vi "Dashboard Main.vi"() -> ()   [LabVIEW 2012]
uses:
  <vilib>/event_ctls.llb/eventvkey.ctl
  <vilib>/Utility/config.llb/Read Key (String).vi
  <vilib>/Utility/config.llb/Read Key (I32).vi
  <vilib>/Utility/config.llb/Write Key (String).vi
  <vilib>/Utility/config.llb/Write Key (I32).vi
  <vilib>/Utility/config.llb/NI_LVConfig.lvlib
  <vilib>/vision/NI_Vision_Development_Module.lvlib
panel:
  out "Battery Value":dbl(slide) scale=0.0..14.0 scale format="%#_2e"
  out "Battery":sgl(graph)
  in  "Camera Settings":T1={"Frate Rate"=30, "Compression"=30, "Size"=1} {"Frate Rate" scale=1.0..30.0; "Size" items=["640x480", "320x240", "160x120"]}
  out "Mode":T2(ring)=enum."Auto Disabled"
  out "Camera IP":string
  out "JS1 Z":dbl(slide) scale=-1.0..1.0 scale format="%#_2e"
  out "JS2 Z":dbl(slide) scale=-1.0..1.0 scale format="%#_2e"
  out "Joystick 1":cluster{"X":dbl, "Y":dbl}[](graph)
  out "Joystick 2":cluster{"X":dbl, "Y":dbl}[](graph)
  out "JS Buttons 1":T3
  out "JS Buttons 2":T3
  out "MotorSlide4":dbl(slide) scale=-1.0..1.0 scale format="%#_2e"
  out "MotorSlide3":dbl(slide) scale=-1.0..1.0 scale format="%#_2e"
  out "MotorSlide2":dbl(slide) scale=-1.0..1.0 scale format="%#_2e"
  in  "MotorName3":string="Front Left"
  in  "MotorName4":string="Front Right"
  in  "MotorName1":string="Rear Left"
  in  "MotorName2":string="Rear Right"
  out "MotorChart4":dbl(graph)
  out "MotorChart3":dbl(graph)
  out "MotorChart2":dbl(graph)
  out "MotorSlide1":dbl(slide) scale=-1.0..1.0 scale format="%#_2e"
  out "MotorChart1":dbl(graph)
  out "Robot IP":string
  in  "Dashboard Tab":enum32{"Operation", "Test", "Checklist"}(tab)
  in  "Checkbox 2":bool
  in  "Checkbox 1":bool
  in  "Slider 1":dbl(slide) scale=0.0..100.0
  in  "Slider":dbl(slide) scale=0.0..100.0 scale format="%#_3g"
  in  "On/Off":bool caption="Solenoid"
  in  "Test Name":u16(ring) items=["Select the test to run...", "Example Test", "-------------------------------", "List of tests is built in robot code.", "Replace with your own automated tests."]
  in  "Test Tree":string(tree)
  in  "Motor":cluster{"Value":dbl, "Enable":bool} {"Value" scale=-1.0..1.0 scale format="%#_3g"}
  out "Progress":T4 {"Test Progress" scale=0.0..100.0}
  in  "Rev/Fwd":cluster{"Forward":bool, "Reverse":bool}
  in  "Ring":u16(ring) items=["Auto", "Fixed indoor", "Fixed outdoor 1", "Fixed outdoor 2", "Fixed fluorescent 1", "Fixed fluorescent 2", "Hold current"]
  in  "Listbox":i32(listbox)
  in  "Viewer":T5(tab)
  out "Mbps":dbl format="%#.1g"
  in  "Enable":bool=TRUE
  in  "DB Camera Config":bool
  out "Mbps":bool
  out "fps":dbl format="%#.1g"
  out "Image Error Message":string="Timeout in Camera Communications"
  out "Camera Image":T6(plugin-control)
  out "Buttons 1":cluster{"1":bool, "2":bool, "3":bool}
  out "Kinect 1":cluster{"X":dbl, "Y":dbl, "Z":dbl} {"X" scale=1.0..-1.0; "Y" scale=1.0..-1.0; "Z" scale=1.0..-1.0}
  out "Buttons 2":cluster{"1":bool, "2":bool, "3":bool}
  out "Kinect 2":cluster{"X":dbl, "Y":dbl, "Z":dbl} {"X" scale=1.0..-1.0; "Y" scale=1.0..-1.0; "Z" scale=1.0..-1.0}
  out "Version":string
  out "Skeleton Picture":picture
  out "Players":i8
  out "Tree":string(tree)
  # "Drive & Motors"
  # "Robot IP:"
  # "Customize by placing controls and indicators here and name to match\nDashboard Variables on robot."
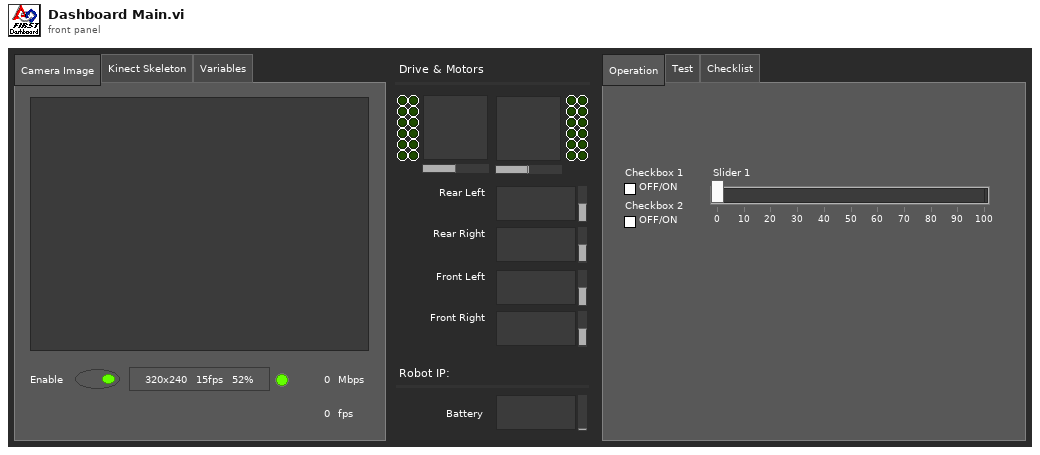
[diagram p1: front panel]
types:
  T1 = cluster{"Frate Rate":i32, "Compression":i32, "Size":u16}
  T2 = enum8{"Tele-Op Disabled", "Tele-Op Enabled", "Auto Disabled", "Auto Enabled", "Test Disabled", "Test Enabled", ""}
  T3 = cluster{bool, bool, bool, bool, bool, bool, bool, bool, bool, bool, bool, bool}
  T4 = cluster{"Test Progress":u8, "Test Progress Text":string}
  T5 = enum32{"Camera Image", "Kinect Skeleton", "Variables"}
  T6 = typedef "IMAQ Image.ctl" = refnum<image>
  T7 = typedef "Image Type" = u32
  T8 = typedef "LVBoundsTypeDef.ctl" = cluster{"Width":u32, "Height":u32}
  T9 = typedef "SkeletonTrackState.ctl" = enum32{"NotTracked", "PositionOnly", "Tracked"}
  T10 = cluster{"TrackingState":u8[], "Position":cluster{"x":sgl, "y":sgl, "z":sgl}, cluster{"x":sgl, "y":sgl, "z":sgl, sgl}[], "TrackState":T9}
  T11 = cluster{cluster{"ScaledToPercentRange":dbl, "ScaledToPercentRange":dbl, "ScaledToPercentRange":dbl}, cluster{bool, bool, bool}}[]
  T12 = cluster{cluster{"ScaledToPercentRange":dbl, "ScaledToPercentRange":dbl, "ScaledToPercentRange":dbl}, cluster{bool, bool, bool}}
  T13 = cluster{"ScaledToPercentRange":dbl, "ScaledToPercentRange":dbl, "ScaledToPercentRange":dbl}
  T14 = typedef "LVRectTypeDef.ctl" = cluster{"Left":i16, "Top":i16, "Right":i16, "Bottom":i16}
  T15 = cluster{"Competition mode":bool, "Robot Link":bool, "Autonomous":bool, "Enabled":bool, "E-Stop":bool, "Simulated":bool, "TestMode":bool, "Docked Window":bool}
  T16 = cluster{"Boolean Array[0]":bool, "Boolean Array[1]":bool, "Boolean Array[2]":bool, "Boolean Array[3]":bool, "Boolean Array[4]":bool, "Boolean Array[5]":bool, "Boolean Array[6]":bool, "Boolean Array[7]":bool, "Boolean Array[8]":bool, "Boolean Array[9]":bool, "Boolean Array[10]":bool, "Boolean Array[11]":bool}
  T17 = typedef "NI_LVConfig.lvlib/Config Data RefNum.ctl" = refnum<k1>
  T18 = typedef "eventvkey.ctl" = enum16{"ASCII", "Enter", "Return", "Shift", "Ctrl", "Alt", "Cmd", "Opt", "Caps", "NumLock", "Clear", "Break", "Up", "Down", "Left", "Right", "Insert", "Delete", "Home", "End", "PageUp", "PageDown", "Escape", "Help", "Pause", "ScrollLock", "F1", "F2", "F3", "F4", "F5", "F6", "F7", "F8", "F9", "F10", "F11", "F12", "F13", "F14", "F15", "F16", "F17", "F18", "F19", "F20", "F21", "F22", "F23", "F24", "Play", "VolumeUp", "VolumeDown", "Mute", "Two Byte Char"}
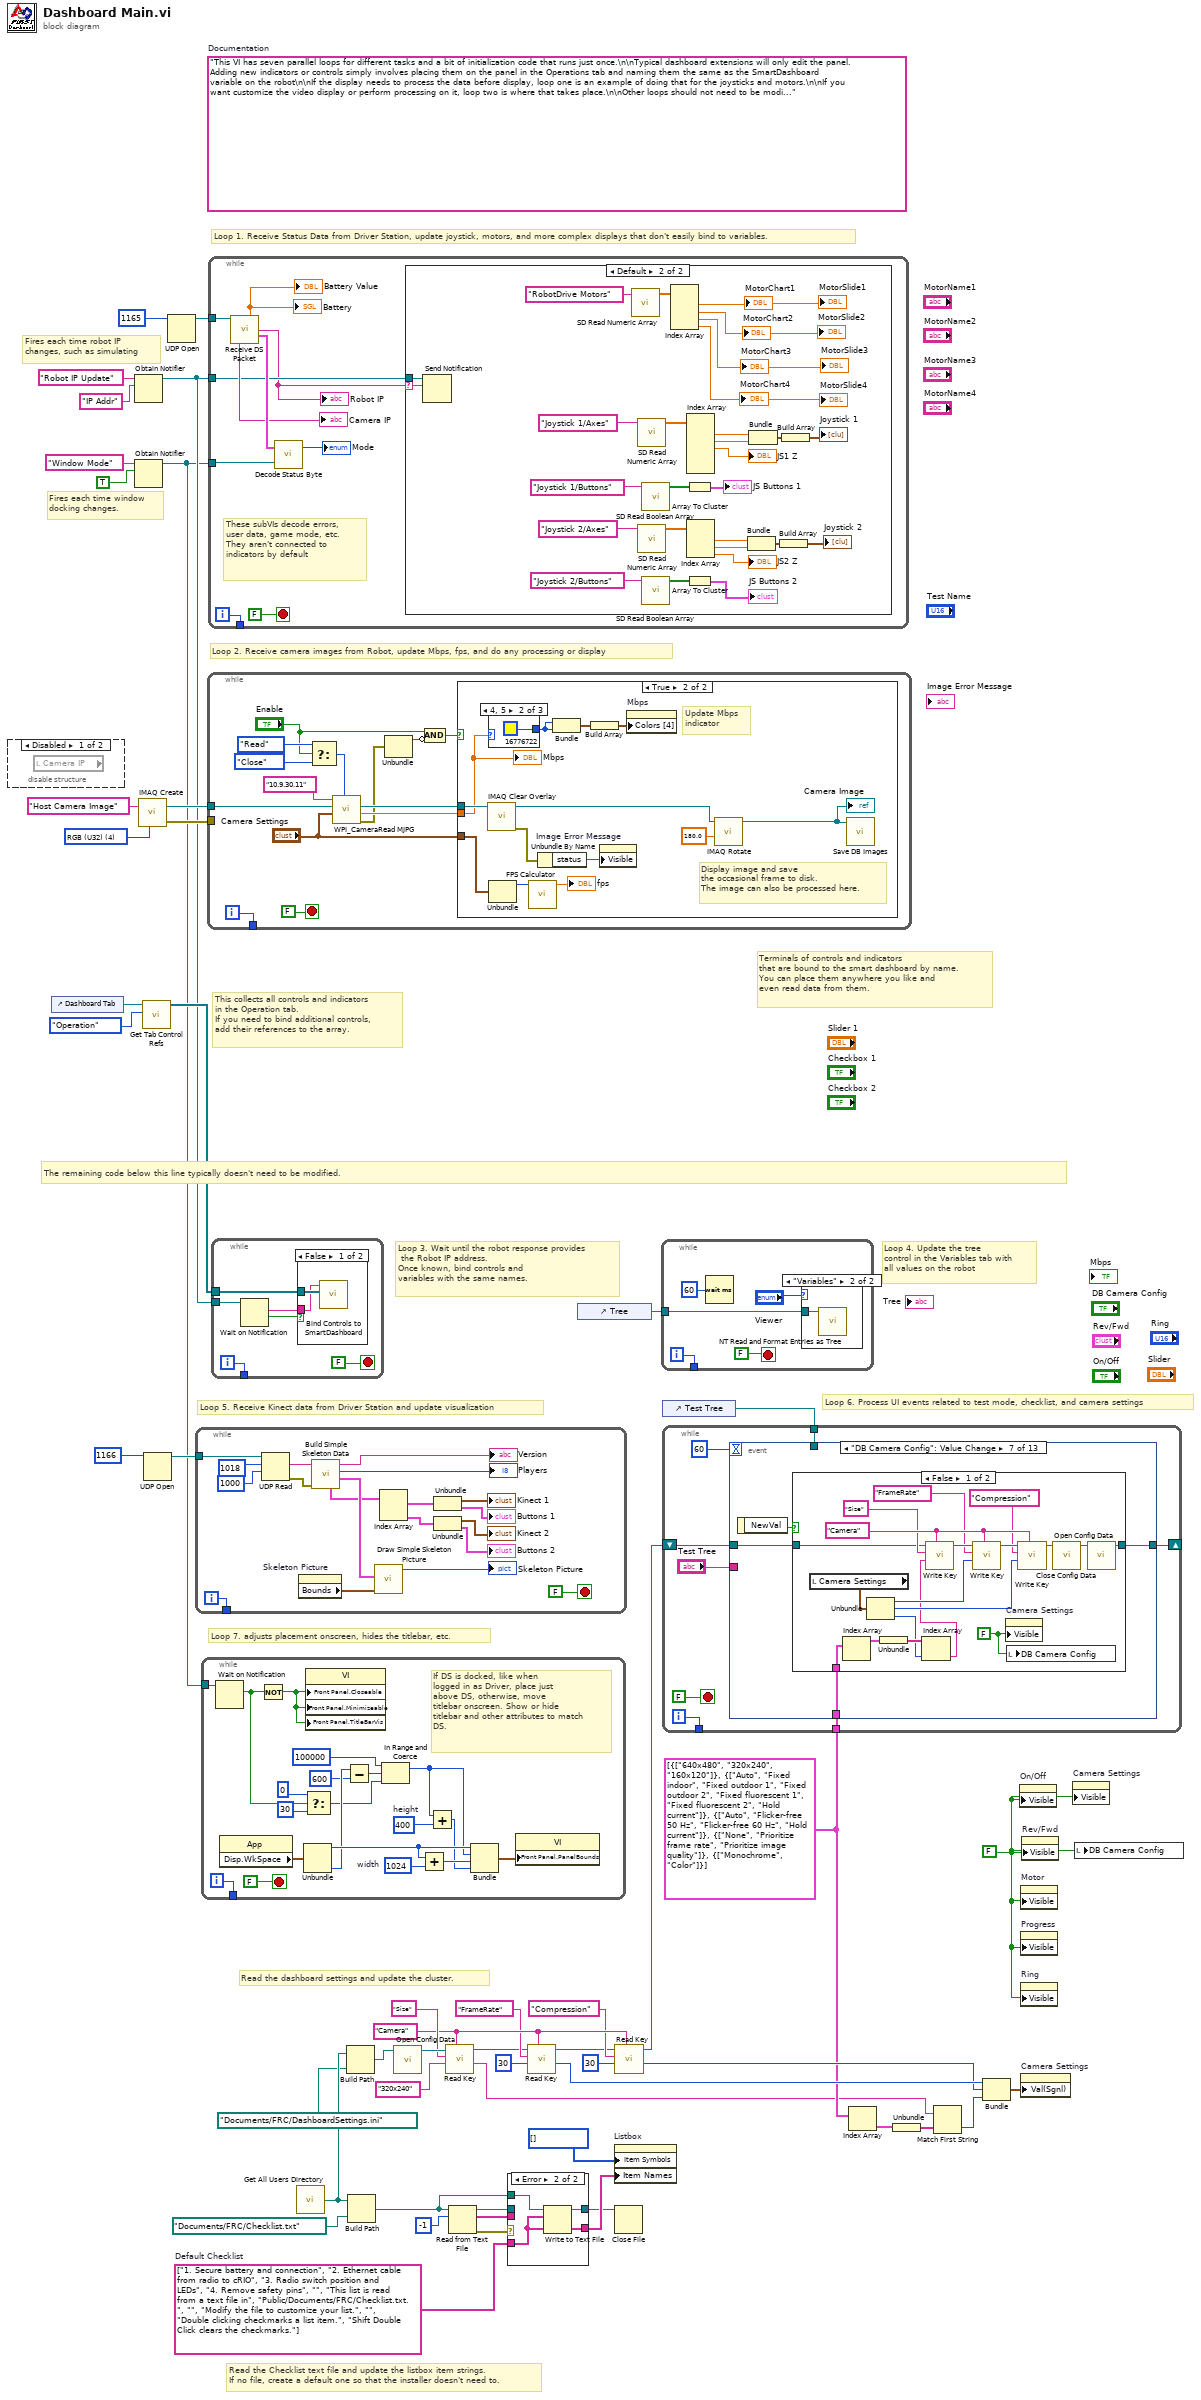
[diagram p0: block diagram]
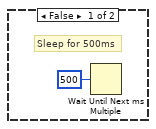
[diagram p4: hidden frame]
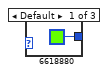
[diagram p5: hidden frame]
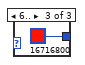
[diagram p6: hidden frame]
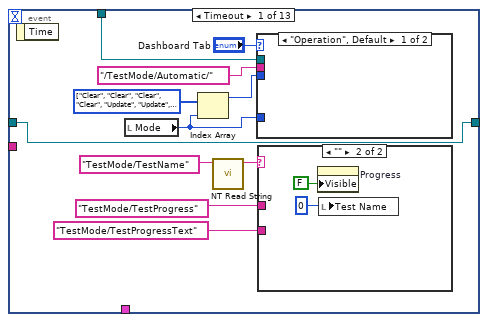
[diagram p8: hidden frame]
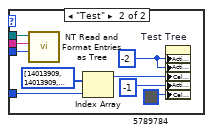
[diagram p9: hidden frame]
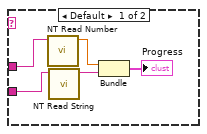
[diagram p10: hidden frame]
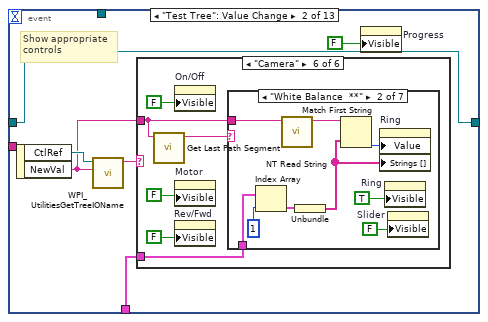
[diagram p11: hidden frame]
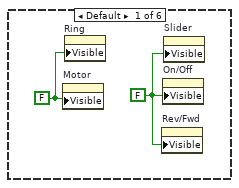
[diagram p12: hidden frame]
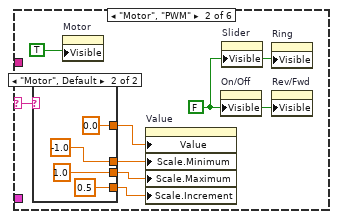
[diagram p13: hidden frame]
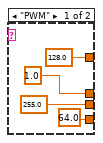
[diagram p14: hidden frame]
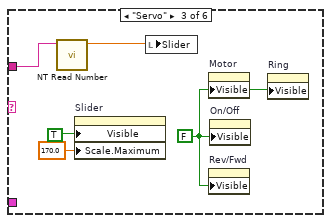
[diagram p15: hidden frame]
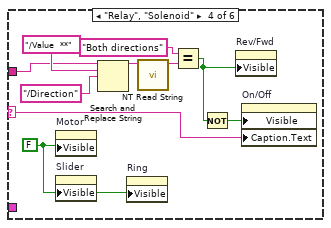
[diagram p16: hidden frame]
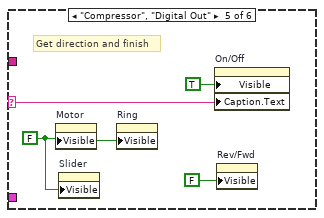
[diagram p17: hidden frame]
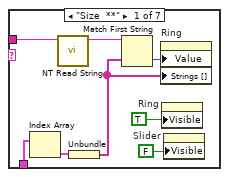
[diagram p18: hidden frame]
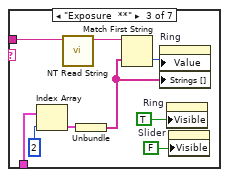
[diagram p19: hidden frame]
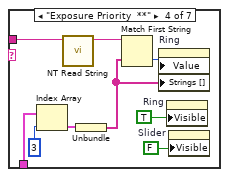
[diagram p20: hidden frame]
diagram:
  w21 = "Camera"
  w13 = cluster{string[]}[] [{["640x480", "320x240", "160x120"]}, {["Auto", "Fixed indoor", "Fixed outdoor 1", "Fixed outdoor 2", "Fixed fluorescent 1", "Fixed fluorescent 2", "Hold current"]}, {["Auto", "Flicker-free 50 Hz", "Flicker-free 60 Hz", "Hold current"]}, {["None", "Prioritize frame rate", "Prioritize image quality"]}, {["Monochrome", "Color"]}]
  w29 = string[] ["1. Secure battery and connection", "2. Ethernet cable from radio to cRIO", "3. Radio switch position and LEDs", "4. Remove safety pins", "", "This list is read from a text file in", "Public/Documents/FRC/Checklist.txt.", "", "Modify the file to customize your list.", "", "Double clicking checkmarks a list item.", "Shift Double Click clears the checkmarks."]  # Default Checklist
  w27 = FALSE ("Visible")
  (unwired) "This VI has seven parallel loops for different tasks and a bit of initialization code that runs just once.\n\nTypical dashboard extensions will only edit the panel. Adding new indicators or controls simply involves placing them on the panel in the Operations tab and naming them the same as the SmartDashboard variable on the robot\n\nIf the display needs to process the data before display, loop one is an example of doing that for the joysticks and motors.\n\nIf you want customize the video display or perform processing on it, loop two is where that takes place.\n\nOther loops should not need to be modified. They are pretty standard, and document the task they perform."  # Documentation
  w50 = T7 4 items=["Grayscale (U8)", "Grayscale (I16)", "Grayscale (SGL)", "Complex (CSG)", "RGB (U32)", "HSL (U32)", "RGB (U64)"] ("Image Type")
  # "Fires each time robot IP\nchanges, such as simulating"
  # "Fires each time window\ndocking changes."
  # "Read the Checklist text file and update the listbox item strings.\nIf no file, create a default one so that the installer doesn't need to."
  # "This collects all controls and indicators\nin the Operation tab.\nIf you need to bind additional controls,\nadd their references to the array."
  # "The remaining code below this line typically doesn't need to be modified."
  # "Loop 6. Process UI events related to test mode, checklist, and camera settings"
  # "Read the dashboard settings and update the cluster."
  # "Terminals of controls and indicators\nthat are bound to the smart dashboard by name.\nYou can place them anywhere you like and\neven read data from them."
  # "Loop 4. Update the tree\ncontrol in the Variables tab with\nall values on the robot"
  # "Loop 3. Wait until the robot response provides\n the Robot IP address.\nOnce known, bind controls and\nvariables with the same names."
  # "Loop 5. Receive Kinect data from Driver Station and update visualization"
  # "Loop 7. adjusts placement onscreen, hides the titlebar, etc."
  # "Loop 1. Receive Status Data from Driver Station, update joystick, motors, and more complex displays that don't easily bind to variables."
  # "Loop 2. Receive camera images from Robot, update Mbps, fps, and do any processing or display"
  n1 = disable-structure shown="Disabled" {
    frame Disabled {
      n2 = local read "Camera IP"() -> ()  [unwired: 1 out]
    }
    frame Enabled {
    }
  }
  n3 = control-ref of="Dashboard Tab"() -> (w43:refnum<vi>)
  n4 = Obtain Notifier(name (unnamed)="Robot IP Update", notification data type="IP Addr" ("name (unnamed)")) -> (notifier out=w40:refnum<notifier>)  [unwired: 2 in, 2 out]
  n5 = Obtain Notifier(name (unnamed)="Window Mode", notification data type=TRUE) -> (notifier out=w33:refnum<notifier>)  [unwired: 2 in, 2 out]
  n6 = call "IMAQ Create"("Image Name"="Host Camera Image", "Image Type"=w50) -> ("New Image"=w48:T6, "error out"=w47:errorcluster)  [unwired: 2 in, 1 out]
  n7 = call <vilib>:"Get Tab Control Refs.vi"("Page Index"=enum32{"Operation", "Test"}."Operation" ("Dashboard Tab"), "TabControl in"=w43) -> ("ControlsOnPage"=w44:refnum<vi>[])  [unwired: 9 in]
  n8 = UDP Open(11:u16 1166 ("port")) -> (port=w45:refnum<k16>)  [unwired: 2 in, 4 out]
  n9 = UDP Open(11:u16 1165 ("port")) -> (port=w51:refnum<k16>)  [unwired: 2 in, 4 out]
  n10 = while {
    tunnel: w45 -> [w69]
    tunnel: [w54] -> _
    i -> [w54]
    stop <- FALSE stop-if-true
    n11 = UDP Read(connection ID=w69, max size (548)=1018 ("bytes to read"), timeout ms (25000)=1000) -> (data out=w63:string, error out=w53:errorcluster)  [unwired: 1 in, 3 out]
    n12 = property on="Skeleton Picture" class="Pict"() -> ("Bounds"=w65:T8)  [unwired: 2 in, 2 out]
    n13 = call "Build Simple Skeleton Data.vi"("error in (no error)"=w53, "data in"=w63) -> ("Skeleton Data"=w64:T10, "NumPlayers"=→"Players":i8, "Version String"=→"Version":string, "Simple Joystick Info"=w61:T11)  [unwired: 5 in, 1 out]
    n14 = call "Draw Simple Skeleton Picture.vi"("Bounds"=w65, "Simple Skeleton"=w64) -> ("new picture out"=→"Skeleton Picture":picture)  [unwired: 9 in]
    n15 = Index Array(array=w61) -> (element #1=w60:T12, element #2=w59:T12)  [unwired: 2 in]
    n16 = Unbundle(w60) -> (→"Kinect 1":T13, →"Buttons 1":cluster{bool, bool, bool})
    n17 = Unbundle(w59) -> (→"Kinect 2":T13, →"Buttons 2":cluster{bool, bool, bool})
  }
  n18 = while {
    tunnel: w33 -> [w90]
    tunnel: [w88] -> _
    i -> [w88]
    stop <- FALSE stop-if-true
    w80 = 1024  # width
    w83 = 400  # height
    # "If DS is docked, like when\nlogged in as Driver, place just\nabove DS, otherwise, move\ntitlebar onscreen. Show or hide\ntitlebar and other attributes to match\nDS."
    n19 = Wait on Notification(notifier=w90) -> (notification=w75:bool)  [unwired: 3 in, 3 out]
    n20 = property class="App"() -> ("Disp.WkSpace"=w86:T14)  [unwired: 2 in, 2 out]
    n21 = Not(x=w75) -> (.not. x?=w89:bool)
    n22 = Unbundle(w86) -> ("Left"=w84:i16, "Bottom"=w81:i16)  [unwired: 2 out]
    n23 = Select(t=0, s=w75, f=30) -> (s? t:f=w74:i32)
    n24 = property class="VI"("Front Panel.Closeable"=w89, "Front Panel.Minimizeable"=w89, "Front Panel.TitleBarVis"=w89) -> ()  [unwired: 2 in, 2 out]
    n25 = Subtract(x=w81, y=600) -> (x-y=w78:i32)
    n26 = In Range and Coerce(upper limit=100000, x=w78, lower limit=w74) -> (coerced(x)=w72:i32)  [unwired: 1 out]
    n27 = Add(x=w84, y=w80) -> (x+y=w85:i32)
    n28 = Add(x=w72, y=w83) -> (x+y=w82:i32)
    n29 = Bundle("Left"=w84, w72, w85, w82) -> (w87:cluster{"Left":i16, i32, i32, i32})  [unwired: 1 out]
    n30 = property class="VI"("Front Panel.PanelBounds"=w87) -> ()  [unwired: 2 in, 2 out]
  }
  n31 = while {
    tunnel: w48 -> [w102]
    tunnel: w47 -> [_]
    tunnel: [w104] -> _
    i -> [w104]
    stop <- FALSE stop-if-true
    n32 = Select(t=enum16{"Read", "Reopen", "Close"}."Read" ("Operation"), s="Enable", f=enum16{"Read", "Reopen", "Close"}."Close" ("Operation")) -> (s? t:f=w97:enum16{"Read", "Reopen", "Close"})
    n33 = call <vilib>:"WPI_CameraRead MJPG.vi"("Operation"=w97, "Camera Settings"="Camera Settings", "Image"=w102, "address"="10.9.30.11") -> ("error out"=w96:errorcluster, "Bandwidth (kbps)"=w100:dbl, "Image Out"=w101:T6)  [unwired: 5 in]
    n34 = Unbundle(w96) -> ("status"=w94:bool)  [unwired: 2 out]
    n35 = Compound Arithmetic op=AND("Enable", invert w94) -> (w93:bool)
    n36 = case shown="True" w93 {
      tunnel: "Camera Settings" -> [_ w111]
      tunnel: w101 -> [_ w114]
      tunnel: w100 -> [_ w113]
      frame False {
        # "Sleep for 500ms"
        n37 = Wait Until Next ms Multiple(millisecond multiple=u32 500) -> ()  [unwired: 1 out]
      }
      frame True {
        # "Display image and save\nthe occasional frame to disk.\nThe image can also be processed here."
        # "Update Mbps\nindicator"
        n38 = call "IMAQ Clear Overlay"("Image"=w114) -> ("error out"=w118:errorcluster, "Image Out"=w109:T6)  [unwired: 2 in, 7 out]
        n39 = case shown="4, 5" w113 {
          tunnel: [u32 6618880 ("Color Box") u32 16776722 ("Color Box") u32 16716800 ("Color Box")] -> w115
          frame Default {
          }
          frame 4, 5 {
          }
          frame 6.. {
          }
        }
        n40 = Unbundle(w111) -> ("Frate Rate"=w110:i32)  [unwired: 2 out]
        n41 = call "FPS Calculator.vi"("Average Count"=w110) -> ("fps"=→"fps":dbl)  [unwired: 10 in]
        n42 = Unbundle By Name(w118) -> ("status"=w119:bool)
        n43 = Bundle("Color Box"=w115, "Color Box"=w115) -> (w117:cluster{"Color Box":u32, "Color Box":u32})  [unwired: 1 out]
        n44 = Build Array(w117) -> (w116:cluster{"Color Box":u32, "Color Box":u32}[])
        n45 = property on="Image Error Message" class="Str"("Visible"=w119) -> ()  [unwired: 2 in, 2 out]
        n46 = property on="Mbps" class="Bool (strict)"("Colors [4]"=w116) -> ()  [unwired: 2 in, 2 out]
        n47 = call "IMAQ Rotate"("Angle (degrees)"=sgl 180.0, "Image Src"=w109) -> ("Image Dst Out"=w107:T6)  [unwired: 8 in, 1 out]
        "Camera Image" <- w107
        n48 = call "Save DB Images.vi"("Image"=w107) -> ()  [unwired: 2 in, 1 out]
        "Mbps" <- w113
      }
    }
  }
  n49 = while {
    tunnel: w51 -> [w130]
    tunnel: w40 -> [w124]
    tunnel: w33 -> [w128]
    tunnel: [w125] -> _
    i -> [w125]
    stop <- FALSE stop-if-true
    # "These subVIs decode errors, user data, game mode, etc.\nThey aren't connected to indicators by default"
    n50 = call "Receive DS Packet.vi"("Recv Socket"=w130) -> ("Battery"=→"Battery" →"Battery Value":sgl, "Robot IP Address"=w123:string, "Status"=w131:T15, "Camera IP Address"=→"Camera IP":string)  [unwired: 1 in, 10 out]
    "Robot IP" <- w123
    n51 = call "Decode Status Byte.vi"("Window Mode Notifier"=w128, "Status"=w131) -> ("Mode"=→"Mode":T2)  [unwired: 1 out]
    n52 = case shown="Default" w123 {
      selector: w123 -> [_ w133]
      tunnel: w124 -> [_ w134]
      frame "0.0.0.0" {
        # "Robot not responding, don't poll the variables"
      }
      frame Default {
        n53 = Send Notification(notification=w133, notifier=w134) -> ()  [unwired: 1 in, 2 out]
        n54 = call <vilib>:"SD Read Numeric Array.vi"("Name"="RobotDrive Motors") -> ("Numeric Array"=w157:dbl[])  [unwired: 8 in, 2 out]
        n55 = call <vilib>:"SD Read Numeric Array.vi"("Name"="Joystick 1/Axes") -> ("Numeric Array"=w150:dbl[])  [unwired: 8 in, 2 out]
        n56 = call <vilib>:"SD Read Numeric Array.vi"("Name"="Joystick 2/Axes") -> ("Numeric Array"=w144:dbl[])  [unwired: 8 in, 2 out]
        n57 = call <vilib>:"SD Read Boolean Array.vi"("Name"="Joystick 1/Buttons") -> ("Boolean Array"=w152:bool[])  [unwired: 8 in, 2 out]
        n58 = call <vilib>:"SD Read Boolean Array.vi"("Name"="Joystick 2/Buttons") -> ("Boolean Array"=w143:bool[])  [unwired: 8 in, 2 out]
        n59 = Index Array(array=w157) -> (element #1=→"MotorChart1" →"MotorSlide1":dbl, element #2=→"MotorSlide2" →"MotorChart2":dbl, element #3=→"MotorChart3" →"MotorSlide3":dbl, element #4=→"MotorChart4" →"MotorSlide4":dbl)  [unwired: 4 in]
        n60 = Array To Cluster(array=w152) -> (cluster=→"JS Buttons 1":T16)
        n61 = Array To Cluster(array=w143) -> (cluster=→"JS Buttons 2":T16)
        n62 = Index Array(array=w150) -> (element #1=w147:dbl, element #2=w148:dbl, element #3=→"JS1 Z":dbl)  [unwired: 6 in, 3 out]
        n63 = Index Array(array=w144) -> (element #1=w139:dbl, element #2=w138:dbl, element #3=→"JS2 Z":dbl)  [unwired: 3 in]
        n64 = Bundle("Numeric"=w139, "Numeric"=w138) -> (w140:cluster{"Numeric":dbl, "Numeric":dbl})  [unwired: 1 in]
        n65 = Bundle("Numeric"=w147, "Numeric"=w148) -> (w146:cluster{"Numeric":dbl, "Numeric":dbl})  [unwired: 1 in]
        n66 = Build Array(w140) -> (→"Joystick 2":cluster{"Numeric":dbl, "Numeric":dbl}[])
        n67 = Build Array(w146) -> (→"Joystick 1":cluster{"Numeric":dbl, "Numeric":dbl}[])
      }
    }
  }
  n68 = while {
    tunnel: w44 -> [w166]
    tunnel: w40 -> [w163]
    tunnel: [w161] -> _
    i -> [w161]
    stop <- FALSE stop-if-true
    n69 = Wait on Notification(notifier=w163) -> (notification=w162:string, timed out?=w164:bool)  [unwired: 3 in, 2 out]
    n70 = case shown="False" w164 {
      tunnel: w166 -> [w168 _]
      tunnel: w162 -> [w167 _]
      frame False {
        n71 = call <vilib>:"Bind Controls to SmartDashboard.vi"("Bound Control Refs"=w168, "Server IP Address"=w167) -> ()  [unwired: 10 in]
      }
      frame True {
      }
    }
  }
  n72 = call "Get All Users Directory.vi"() -> ("All User Path"=w26:path)
  n73 = Build Path(base path=w26, name or relative path=path "Documents/FRC/DashboardSettings.ini") -> (appended path=w25:path)
  n74 = Build Path(base path=w26, name or relative path=path "Documents/FRC/Checklist.txt") -> (appended path=w30:path)
  n75 = call <vilib>:"Open Config Data.vi"("configuration file path"=w25) -> ("refnum"=w24:T17)  [unwired: 8 in, 2 out]
  n76 = call-poly <vilib>:"Read Key.vi"("section"=w21, "default value"="320x240", "key"="Size", "refnum"=w24) -> ("value"=w11:string, "refnum out"=w6:T17)  [unwired: 2 in, 4 out]
  n77 = Read from Text File(file (use dialog)=w30, count=-1 ("timeout ms (25000)")) -> (refnum out=w8:refnum<file>, text=w31:string[], error out=w32:errorcluster)  [unwired: 2 in, 1 out]
  n78 = case shown="Error" w32 {
    tunnel: w31 -> [w170 _]
    tunnel: [w170 w172] -> w28
    tunnel: w29 -> [_ w172]
    tunnel: w30 -> [_ w173]
    tunnel: [w169 w171] -> w7
    tunnel: w8 -> [w169 _]
    frame No Error {
    }
    frame Error {
      n79 = Write to Text File(file (use dialog)=w173, text=w172) -> (refnum out=w171:refnum<file>)  [unwired: 2 in, 2 out]
    }
  }
  n80 = call-poly <vilib>:"Read Key.vi"("section"=w21, "default value"=30, "key"="FrameRate", "refnum"=w6) -> ("value"=w16:i32, "refnum out"=w5:T17)  [unwired: 1 in, 5 out]
  n81 = control-ref of="Tree"() -> (w2:refnum<vi>)
  n82 = property on="Listbox" class="LstBox (strict)"("Item Symbols"=i32[] [], "Item Names"=w28) -> ()  [unwired: 2 in, 2 out]
  n83 = Close File(refnum=w7) -> ()  [unwired: 1 in, 2 out]
  n84 = call-poly <vilib>:"Read Key.vi"("section"=w21, "default value"=30, "key"="Compression", "refnum"=w5) -> ("value"=w15:i32, "refnum out"=w3:T17)  [unwired: 1 in, 5 out]
  n85 = while {
    tunnel: [w175] -> _
    tunnel: w2 -> [w174]
    i -> [w175]
    stop <- FALSE stop-if-true
    n86 = Wait (ms)(milliseconds to wait=u32 60) -> ()  [unwired: 1 out]
    n87 = case shown="\"Variables\"" "Viewer" {
      tunnel: w174 -> [_ w179]
      frame Default {
      }
      frame "Variables" {
        n88 = call <vilib>:"NT Read and Format Entries as Tree.vi"("Tree Refnum"=w179) -> ()  [unwired: 9 in, 2 out]
      }
    }
  }
  n89 = control-ref of="Test Tree"() -> (w1:refnum<vi>)
  n90 = while {
    tunnel: w13 -> [w184]
    shift-right: [w183] -> _
    shift-left: w3 -> [w182]
    tunnel: [w181] -> _
    tunnel: w1 -> [w180]
    i -> [w181]
    stop <- FALSE stop-if-true
    n91 = event shown="[6] \"DB Camera Config\": Value Change" {
      selector: _ -> [_ _ _ _ _ _ _ _ _ _ _ _ _]
      dyn-events: _ -> [_ _ _ _ _ _ _ _ _ _ _ _ _]
      timeout: u32 60 ("milliseconds to wait") -> [_ _ _ _ _ _ _ _ _ _ _ _ _]
      tunnel: w180 -> [w194 _ _ _ _ _ _ _ _ _ _ _ _]
      tunnel: "Test Tree" -> [_ _ _ _ _ _ _ _ w388 w396 w398 w402 w410]
      tunnel: w184 -> [_ w216 _ _ _ _ w352 w382 _ _ _ _ _]
      tunnel: [w188 w215 _ w318 w326 w338 w351 w375 w387 w394 w397 w401 w409] -> w183
      tunnel: w182 -> [w188 w215 _ w318 w326 w338 w350 w375 w387 w394 w397 w401 w409]
      event Timeout {
        w193 = enum16{"Update", "Clear"}[] [enum."Clear", enum."Clear", enum."Clear", enum."Clear", enum."Update", enum."Update", enum."Clear"] items=["Update", "Clear"]
        n92 = event-data() -> ()  [unwired: 1 in, 1 out]
        n93 = local read "Mode"() -> (w191:T2)
        n94 = Index Array(array=w193, index=w191) -> (element=w192:enum16{"Update", "Clear"})
        n95 = call <vilib>:"NT Read String.vi"("Name"="TestMode/TestName") -> ("String"=w197:string)  [unwired: 9 in, 1 out]
        n96 = case shown="\"Operation\", Default" "Dashboard Tab" {
          tunnel: w194 -> [_ w207]
          tunnel: "/TestMode/Automatic/" ("Name Pattern") -> [_ w206]
          tunnel: w192 -> [_ w205]
          tunnel: w191 -> [_ w203]
          frame "Operation", Default {
          }
          frame "Test" {
            w202 = -2 ("Active Item:Row Number")
            n97 = call <vilib>:"NT Read and Format Entries as Tree.vi"("Operation"=w205, "Name Pattern"=w206, "Tree Refnum"=w207) -> ()  [unwired: 7 in, 2 out]
            n98 = Index Array(array=u32[] [14013909, 14013909, 14013909, 14013909, 14013909, 16777215, 14013909], index=w203) -> (element=w201:u32)
            n99 = property on="Test Tree" class="Tree (strict)"("Active Item Row Number"=w202, "ActiveColNum"=w202, "CellBG"=w201, "Active Item Row Number"=-1 ("Active Item:Row Number"), "CellBG"=u32 5789784 ("Color Box")) -> ()  [unwired: 2 in, 2 out]
          }
        }
        n100 = case shown="\"\"" w197 {
          tunnel: "TestMode/TestProgress" ("Name") -> [w209 _]
          tunnel: "TestMode/TestProgressText" ("Name") -> [w208 _]
          frame Default {
            n101 = call <vilib>:"NT Read Number.vi"("Name"=w209) -> ("Numeric"=w210:dbl)  [unwired: 9 in, 1 out]
            n102 = call <vilib>:"NT Read String.vi"("Name"=w208) -> ("String"=w211:string)  [unwired: 9 in, 1 out]
            n103 = Bundle("Numeric"=w210, "String"=w211) -> (→"Progress":cluster{"Numeric":dbl, "String":string})  [unwired: 1 in]
          }
          frame "" {
            n104 = property on="Progress" class="Clust (strict)"("Visible"=FALSE) -> ()  [unwired: 2 in, 2 out]
            n105 = local write "Test Name"(u16 0) -> ()
          }
        }
      }
      event "Test Tree": Value Change {
        # "Show appropriate\ncontrols"
        n106 = event-data() -> ("CtlRef"=w219:refnum<vi>, "NewVal"=w217:string)  [unwired: 1 in]
        n107 = call <vilib>:"WPI_UtilitiesGetTreeIOName.vi"("NewVal"=w217, "TreeControl in"=w219) -> ("I/O Name"=w220:string)  [unwired: 9 in]
        n108 = case shown="\"Camera\"" w220 {
          selector: w220 -> [_ w227 _ w245 w254 _]
          tunnel: w217 -> [_ _ w242 w244 _ w261]
          tunnel: w216 -> [_ _ _ _ _ w260]
          frame Default {
            w222 = FALSE ("Visible")
            w221 = FALSE ("Visible")
            n109 = property on="Motor" class="Clust (strict)"("Visible"=w221) -> ()  [unwired: 2 in, 2 out]
            n110 = property on="Ring" class="Ring (strict)"("Visible"=w221) -> ()  [unwired: 2 in, 2 out]
            n111 = property on="Rev/Fwd" class="Clust (strict)"("Visible"=w222) -> ()  [unwired: 2 in, 2 out]
            n112 = property on="On/Off" class="Bool (strict)"("Visible"=w222) -> ()  [unwired: 2 in, 2 out]
            n113 = property on="Slider" class="Slide (strict)"("Visible"=w222) -> ()  [unwired: 2 in, 2 out]
          }
          frame "Motor", "PWM" {
            w228 = FALSE ("Visible")
            n114 = case shown="\"Motor\", Default" w227 {
              tunnel: [1.0 ("Value") -1.0 ("Value")] -> w226
              tunnel: [255.0 ("Value") 1.0 ("Value")] -> w225
              tunnel: [128.0 ("Value") 0.0 ("Value")] -> w224
              tunnel: [64.0 ("Value") 0.5 ("Value")] -> w223
              frame "PWM" {
              }
              frame "Motor", Default {
              }
            }
            n115 = property on="Motor" class="Clust (strict)"("Visible"=TRUE) -> ()  [unwired: 2 in, 2 out]
            n116 = property on="Value" class="Slide (strict)"("Value"=w224, "Scale.Minimum"=w226, "Scale.Maximum"=w225, "Scale.Increment"=w223) -> ()  [unwired: 2 in, 2 out]
            n117 = property on="On/Off" class="Bool (strict)"("Visible"=w228) -> ()  [unwired: 2 in, 2 out]
            n118 = property on="Slider" class="Slide (strict)"("Visible"=w228) -> ()  [unwired: 2 in, 2 out]
            n119 = property on="Ring" class="Ring (strict)"("Visible"=w228) -> ()  [unwired: 2 in, 2 out]
            n120 = property on="Rev/Fwd" class="Clust (strict)"("Visible"=w228) -> ()  [unwired: 2 in, 2 out]
          }
          frame "Servo" {
            w240 = FALSE ("Visible")
            n121 = call <vilib>:"NT Read Number.vi"("Name"=w242) -> ("Numeric"=w241:dbl)  [unwired: 9 in, 1 out]
            n122 = property on="Slider" class="Slide (strict)"("Visible"=TRUE, "Scale.Maximum"=170.0 ("Scale.Range:Maximum")) -> ()  [unwired: 2 in, 2 out]
            n123 = local write "Slider"(w241) -> ()
            n124 = property on="Motor" class="Clust (strict)"("Visible"=w240) -> ()  [unwired: 2 in, 2 out]
            n125 = property on="Rev/Fwd" class="Clust (strict)"("Visible"=w240) -> ()  [unwired: 2 in, 2 out]
            n126 = property on="On/Off" class="Bool (strict)"("Visible"=w240) -> ()  [unwired: 2 in, 2 out]
            n127 = property on="Ring" class="Ring (strict)"("Visible"=w240) -> ()  [unwired: 2 in, 2 out]
          }
          frame "Relay", "Solenoid" {
            w243 = FALSE ("Visible")
            n128 = property on="Motor" class="Clust (strict)"("Visible"=w243) -> ()  [unwired: 2 in, 2 out]
            n129 = property on="Slider" class="Slide (strict)"("Visible"=w243) -> ()  [unwired: 2 in, 2 out]
            n130 = Search and Replace String(input string=w244, search string="/Value  **", replace string="/Direction") -> (result string=w250:string)  [unwired: 5 in, 3 out]
            n131 = property on="Ring" class="Ring (strict)"("Visible"=w243) -> ()  [unwired: 2 in, 2 out]
            n132 = call <vilib>:"NT Read String.vi"("Name"=w250) -> ("String"=w248:string)  [unwired: 9 in, 1 out]
            n133 = Equal?(x="Both directions", y=w248) -> (x = y?=w246:bool)
            n134 = Not(x=w246) -> (.not. x?=w247:bool)
            n135 = property on="Rev/Fwd" class="Clust (strict)"("Visible"=w246) -> ()  [unwired: 2 in, 2 out]
            n136 = property on="On/Off" class="Bool (strict)"("Visible"=w247, "Caption.Text"=w245) -> ()  [unwired: 2 in, 2 out]
          }
          frame "Compressor", "Digital Out" {
            w253 = FALSE ("Visible")
            # "Get direction and finish"
            n137 = property on="Motor" class="Clust (strict)"("Visible"=w253) -> ()  [unwired: 2 in, 2 out]
            n138 = property on="Slider" class="Slide (strict)"("Visible"=w253) -> ()  [unwired: 2 in, 2 out]
            n139 = property on="Ring" class="Ring (strict)"("Visible"=w253) -> ()  [unwired: 2 in, 2 out]
            n140 = property on="On/Off" class="Bool (strict)"("Visible"=TRUE, "Caption.Text"=w254) -> ()  [unwired: 2 in, 2 out]
            n141 = property on="Rev/Fwd" class="Clust (strict)"("Visible"=FALSE) -> ()  [unwired: 2 in, 2 out]
          }
          frame "Camera" {
            n142 = call <vilib>:"Get Last Path Segment.vi"("String in"=w261) -> ("String out"=w262:string)  [unwired: 10 in]
            n143 = property on="On/Off" class="Bool (strict)"("Visible"=FALSE) -> ()  [unwired: 2 in, 2 out]
            n144 = property on="Motor" class="Clust (strict)"("Visible"=FALSE) -> ()  [unwired: 2 in, 2 out]
            n145 = property on="Rev/Fwd" class="Clust (strict)"("Visible"=FALSE) -> ()  [unwired: 2 in, 2 out]
            n146 = case shown="\"White Balance  **\"" w262 {
              tunnel: w261 -> [w268 w277 w286 w295 w304 _ w310]
              tunnel: w260 -> [w266 w274 w283 w292 w301 _ _]
              frame "Size  **" {
                n147 = Index Array(array=w266) -> (element=w265:cluster{string[]})  [unwired: 1 in]
                n148 = call <vilib>:"NT Read String.vi"("Name"=w268) -> ("String"=w267:string)  [unwired: 9 in, 1 out]
                n149 = Unbundle(w265) -> (w263:string[])
                n150 = Match First String(2:w263, 3:w267) -> (0:w264:i32)  [unwired: 1 out]
                n151 = property on="Ring" class="Ring (strict)"("Value"=w264, "Strings []"=w263) -> ()  [unwired: 2 in, 2 out]
                n152 = property on="Ring" class="Ring (strict)"("Visible"=TRUE) -> ()  [unwired: 2 in, 2 out]
                n153 = property on="Slider" class="Slide (strict)"("Visible"=FALSE) -> ()  [unwired: 2 in, 2 out]
              }
              frame "White Balance  **" {
                n154 = Index Array(array=w274, index=1) -> (element=w275:cluster{string[]})
                n155 = call <vilib>:"NT Read String.vi"("Name"=w277) -> ("String"=w276:string)  [unwired: 9 in, 1 out]
                n156 = Unbundle(w275) -> (w272:string[])
                n157 = Match First String(2:w272, 3:w276) -> (0:w271:i32)  [unwired: 1 out]
                n158 = property on="Ring" class="Ring (strict)"("Value"=w271, "Strings []"=w272) -> ()  [unwired: 2 in, 2 out]
                n159 = property on="Ring" class="Ring (strict)"("Visible"=TRUE) -> ()  [unwired: 2 in, 2 out]
                n160 = property on="Slider" class="Slide (strict)"("Visible"=FALSE) -> ()  [unwired: 2 in, 2 out]
              }
              frame "Exposure  **" {
                n161 = Index Array(array=w283, index=2) -> (element=w284:cluster{string[]})
                n162 = call <vilib>:"NT Read String.vi"("Name"=w286) -> ("String"=w285:string)  [unwired: 9 in, 1 out]
                n163 = Unbundle(w284) -> (w280:string[])
                n164 = Match First String(2:w280, 3:w285) -> (0:w281:i32)  [unwired: 1 out]
                n165 = property on="Ring" class="Ring (strict)"("Value"=w281, "Strings []"=w280) -> ()  [unwired: 2 in, 2 out]
                n166 = property on="Ring" class="Ring (strict)"("Visible"=TRUE) -> ()  [unwired: 2 in, 2 out]
                n167 = property on="Slider" class="Slide (strict)"("Visible"=FALSE) -> ()  [unwired: 2 in, 2 out]
              }
              frame "Exposure Priority  **" {
                n168 = Index Array(array=w292, index=3) -> (element=w293:cluster{string[]})
                n169 = call <vilib>:"NT Read String.vi"("Name"=w295) -> ("String"=w294:string)  [unwired: 9 in, 1 out]
                n170 = Unbundle(w293) -> (w289:string[])
                n171 = Match First String(2:w289, 3:w294) -> (0:w290:i32)  [unwired: 1 out]
                n172 = property on="Ring" class="Ring (strict)"("Value"=w290, "Strings []"=w289) -> ()  [unwired: 2 in, 2 out]
                n173 = property on="Ring" class="Ring (strict)"("Visible"=TRUE) -> ()  [unwired: 2 in, 2 out]
                n174 = property on="Slider" class="Slide (strict)"("Visible"=FALSE) -> ()  [unwired: 2 in, 2 out]
              }
              frame "Color Enable  **" {
                n175 = Index Array(array=w301, index=4) -> (element=w302:cluster{string[]})
                n176 = call <vilib>:"NT Read String.vi"("Name"=w304) -> ("String"=w303:string)  [unwired: 9 in, 1 out]
                n177 = Unbundle(w302) -> (w298:string[])
                n178 = Match First String(2:w298, 3:w303) -> (0:w299:i32)  [unwired: 1 out]
                n179 = property on="Ring" class="Ring (strict)"("Value"=w299, "Strings []"=w298) -> ()  [unwired: 2 in, 2 out]
                n180 = property on="Ring" class="Ring (strict)"("Visible"=TRUE) -> ()  [unwired: 2 in, 2 out]
                n181 = property on="Slider" class="Slide (strict)"("Visible"=FALSE) -> ()  [unwired: 2 in, 2 out]
              }
              frame Default {
                n182 = property on="Ring" class="Ring (strict)"("Visible"=FALSE) -> ()  [unwired: 2 in, 2 out]
                n183 = property on="Slider" class="Slide (strict)"("Visible"=FALSE) -> ()  [unwired: 2 in, 2 out]
              }
              frame "Brightness  **", "Color Level  **", "Compression  **", "FPS  **", "Sharpness  **" {
                n184 = call <vilib>:"NT Read Number.vi"("Name"=w310) -> ("Numeric"=w309:dbl)  [unwired: 9 in, 1 out]
                n185 = local write "Slider"(w309) -> ()
                n186 = property on="Slider" class="Slide (strict)"("Visible"=TRUE, "Scale.Maximum"=100.0 ("Scale.Range:Maximum")) -> ()  [unwired: 2 in, 2 out]
                n187 = property on="Ring" class="Ring (strict)"("Visible"=FALSE) -> ()  [unwired: 2 in, 2 out]
              }
            }
          }
        }
        n188 = property on="Progress" class="Clust (strict)"("Visible"=FALSE) -> ()  [unwired: 2 in, 2 out]
      }
      event "Test Name": Mouse Enter {
        # "Populate the ring with the list of tests"
        n189 = event-data() -> ()  [unwired: 1 in, 1 out]
        n190 = call <vilib>:"NT Read String Array.vi"("Name"="TestMode/TestList") -> ("String Array"=w317:string[])  [unwired: 9 in, 1 out]
        n191 = Build Array (concatenate)("Select the test to run...", w317) -> (w316:string[])
        n192 = property on="Test Name" class="Ring (strict)"("Strings []"=w316) -> ()  [unwired: 2 in, 2 out]
      }
      event "Test Name": Value Change {
        w319 = FALSE ("Visible")
        # "Tell the robot the test name to run"
        n193 = event-data() -> ("NewVal"=w323:u16)  [unwired: 1 in]
        n194 = property on="Test Name" class="Ring (strict)"() -> ("Strings []"=w324:string[])  [unwired: 2 in, 2 out]
        n195 = local write "Progress"(T4 {"Test Progress"=0, "Test Progress Text"=""} ("Progress")) -> ()
        n196 = Index Array(array=w324, index=w323) -> (element=w322:string)
        n197 = call <vilib>:"NT Write String.vi"("String"=w322, "Name"="TestMode/TestName") -> ()  [unwired: 9 in, 1 out]
        n198 = property on="Progress" class="Clust (strict)"("Visible"=TRUE) -> ()  [unwired: 2 in, 2 out]
        n199 = property on="Motor" class="Clust (strict)"("Visible"=w319) -> ()  [unwired: 2 in, 2 out]
        n200 = property on="Slider" class="Slide (strict)"("Visible"=w319) -> ()  [unwired: 2 in, 2 out]
        n201 = property on="On/Off" class="Bool (strict)"("Visible"=w319) -> ()  [unwired: 2 in, 2 out]
        n202 = property on="Rev/Fwd" class="Clust (strict)"("Visible"=w319) -> ()  [unwired: 2 in, 2 out]
        n203 = property on="Ring" class="Ring (strict)"("Visible"=w319) -> ()  [unwired: 2 in, 2 out]
      }
      event "Listbox": Double Click {
        n204 = event-data() -> ("PlatMods.Shift"=w327:bool, "Row"=w329:i32)  [unwired: 1 in]
        n205 = case shown="False" w327 {
          tunnel: w329 -> [w333 _]
          tunnel: 1 -> [w332 _]
          frame False {
            n206 = property on="Listbox" class="LstBox (strict)"() -> ("Item Symbols"=w331:i32[])  [unwired: 2 in, 2 out]
            n207 = Replace Array Subset(array=w331, new element=w332, index=w333) -> (w330:i32[])
            n208 = property on="Listbox" class="LstBox (strict)"("Item Symbols"=w330) -> ()  [unwired: 2 in, 2 out]
          }
          frame True {
            w334 = 0 ("Top Row")
            n209 = property on="Listbox" class="LstBox (strict)"() -> ("Number of Rows"=w336:u32)  [unwired: 2 in, 2 out]
            n210 = Initialize Array(0, w336) -> (w335:i32[])
            n211 = property on="Listbox" class="LstBox (strict)"("Top Row"=w334, "Value"=w334, "Item Symbols"=w335) -> ()  [unwired: 2 in, 2 out]
          }
        }
      }
      event "Listbox": Key Down {
        n212 = event-data() -> ("VKey"=w340:T18)  [unwired: 1 in]
        n213 = case shown="\"Left\", \"Right\"" w340 {
          selector: w340 -> [w345 _]
          tunnel: eventvkey."Left" ("VKey") -> [w343 _]
          frame "Left", "Right" {
            n214 = Equal?(x=w343, y=w345) -> (x = y?=w344:bool)
            n215 = Select(t=0, s=w344, f=1) -> (s? t:f=w346:i32)
            n216 = property on="Listbox" class="LstBox (strict)"() -> ("Item Symbols"=w349:i32[])  [unwired: 2 in, 2 out]
            n217 = Replace Array Subset(array=w349, new element=w346, index="Listbox") -> (w348:i32[])
            n218 = property on="Listbox" class="LstBox (strict)"("Item Symbols"=w348) -> ()  [unwired: 2 in, 2 out]
          }
          frame Default {
          }
        }
      }
      event "DB Camera Config": Value Change {
        n219 = event-data() -> ("NewVal"=w353:bool)  [unwired: 1 in]
        n220 = case shown="False" w353 {
          tunnel: w352 -> [w362 _]
          tunnel: [w355 w373] -> w351
          tunnel: w350 -> [w354 w373]
          frame False {
            w369 = "Camera"
            w372 = FALSE ("Visible")
            n221 = local read "Camera Settings"() -> (w361:T1)
            n222 = Index Array(array=w362) -> (element=w365:cluster{string[]})  [unwired: 1 in]
            n223 = Unbundle(w361) -> ("Frate Rate"=w360:i32, "Compression"=w359:i32, "Size"=w363:u16)
            n224 = Unbundle(w365) -> (w364:string[])
            n225 = Index Array(array=w364, index=w363) -> (element=w358:string)
            n226 = call-poly <vilib>:"Write Key.vi"("section"=w369, "value"=w358, "key"="Size", "refnum"=w354) -> ("refnum out"=w371:T17)  [unwired: 2 in, 5 out]
            n227 = call-poly <vilib>:"Write Key.vi"("section"=w369, "value"=w360, "key"="FrameRate", "refnum"=w371) -> ("refnum out"=w370:T17)  [unwired: 1 in, 6 out]
            n228 = property on="Camera Settings" class="Clust (strict)"("Visible"=w372) -> ()  [unwired: 2 in, 2 out]
            n229 = local write "DB Camera Config"(w372) -> ()
            n230 = call-poly <vilib>:"Write Key.vi"("section"=w369, "value"=w359, "key"="Compression", "refnum"=w370) -> ("refnum out"=w356:T17)  [unwired: 1 in, 6 out]
            n231 = call <vilib>:"Close Config Data.vi"("refnum"=w356) -> ("file path"=w357:path)  [unwired: 2 in, 8 out]
            n232 = call <vilib>:"Open Config Data.vi"("configuration file path"=w357) -> ("refnum"=w355:T17)  [unwired: 8 in, 2 out]
          }
          frame True {
            n233 = property on="Camera Settings" class="Clust (strict)"("Visible"=TRUE) -> ()  [unwired: 2 in, 2 out]
          }
        }
      }
      event "Camera Settings": Value Change {
        n234 = event-data() -> ("NewVal"=w386:T1)  [unwired: 1 in]
        n235 = Index Array(array=w382) -> (element=w381:cluster{string[]})  [unwired: 1 in]
        n236 = Unbundle(w386) -> ("Frate Rate"=w377:i32, "Compression"=w376:i32, "Size"=w379:u16)
        n237 = Unbundle(w381) -> (w380:string[])
        n238 = Index Array(array=w380, index=w379) -> (element=w378:string)
        n239 = Format Into String(format string="%s   %dfps   %d%%", w378, w377, w376) -> (resulting string=w383:string)  [unwired: 2 in, 1 out]
        n240 = Build Array(w383) -> (w384:string[])
        n241 = property on="DB Camera Config" class="Bool (strict)"("Strings [4]"=w384) -> ()  [unwired: 2 in, 2 out]
      }
      event "Motor.Enable": Value Change {
        n242 = event-data() -> ("NewVal"=w392:bool)  [unwired: 1 in]
        n243 = Unbundle("Motor") -> ("Value"=w391:dbl)  [unwired: 1 out]
        n244 = Select(t=w391, s=w392, f=0.0) -> (s? t:f=w389:dbl)
        n245 = call <vilib>:"NT Write Number.vi"("Numeric"=w389, "Name"=w388) -> ()  [unwired: 9 in, 1 out]
      }
      event "Slider": Value Change {
        n246 = event-data() -> ("NewVal"=w395:dbl)  [unwired: 1 in]
        n247 = call <vilib>:"NT Write Number.vi"("Numeric"=w395, "Name"=w396) -> ()  [unwired: 9 in, 1 out]
      }
      event "On/Off": Value Change {
        n248 = event-data() -> ("NewVal"=w400:bool)  [unwired: 1 in]
        n249 = Boolean To (0,1)(Boolean=w400) -> (0, 1=w399:i16)
        n250 = call <vilib>:"NT Write Number.vi"("Numeric"=w399, "Name"=w398) -> ()  [unwired: 9 in, 1 out]
      }
      event "Rev/Fwd": Value Change {
        n251 = event-data() -> ("NewVal.Forward"=w408:bool, "NewVal.Reverse"=w407:bool)  [unwired: 1 in]
        n252 = Boolean To (0,1)(Boolean=w408) -> (0, 1=w404:i16)
        n253 = Boolean To (0,1)(Boolean=w407) -> (0, 1=w406:i16)
        n254 = Negate(x=w406) -> (-x=w405:i16)
        n255 = Add(x=w404, y=w405) -> (x+y=w403:i16)
        n256 = call <vilib>:"NT Write Number.vi"("Numeric"=w403, "Name"=w402) -> ()  [unwired: 9 in, 1 out]
      }
      event "Ring": Value Change {
        n257 = event-data() -> ("NewVal"=w412:u16)  [unwired: 1 in]
        n258 = property on="Ring" class="Ring (strict)"() -> ("Strings []"=w413:string[])  [unwired: 2 in, 2 out]
        n259 = Index Array(array=w413, index=w412) -> (element=w411:string)
        n260 = call <vilib>:"NT Write String.vi"("String"=w411, "Name"=w410) -> ()  [unwired: 9 in, 1 out]
      }
    }
  }
  n261 = Index Array(array=w13) -> (element=w14:cluster{string[]})  [unwired: 1 in]
  n262 = Unbundle(w14) -> (w12:string[])
  n263 = Match First String(2:w12, 3:w11) -> (0:w10:i32)  [unwired: 1 out]
  n264 = Bundle("value"=w16, "value"=w15, "index"=w10) -> (w4:cluster{"value":i32, "value":i32, "index":i32})  [unwired: 1 out]
  n265 = property on="On/Off" class="Bool (strict)"("Visible"=w27) -> ()  [unwired: 2 in, 2 out]
  n266 = property on="Motor" class="Clust (strict)"("Visible"=w27) -> ()  [unwired: 2 in, 2 out]
  n267 = property on="Progress" class="Clust (strict)"("Visible"=w27) -> ()  [unwired: 2 in, 2 out]
  n268 = property on="Ring" class="Ring (strict)"("Visible"=w27) -> ()  [unwired: 2 in, 2 out]
  n269 = property on="Camera Settings" class="Clust (strict)"("Val(Sgnl)"=w4) -> ()  [unwired: 2 in, 2 out]
  n270 = property on="Rev/Fwd" class="Clust (strict)"("Visible"=w27) -> ()  [unwired: 2 in, 2 out]
  n271 = property on="Camera Settings" class="Clust (strict)"("Visible"=w27) -> ()  [unwired: 2 in, 2 out]
  n272 = local write "DB Camera Config"(w27) -> ()
